vi "Set_Dark.vi"(8 "error in (no error)":errorcluster, 10 "Dark":dbl, 11 "Thorlabs_PM100D in":refnum<class "Thorlabs_PM100D.lvclass">) -> (0 "error out":errorcluster, 3 "Thorlabs_PM100D out":refnum<class "Thorlabs_PM100D.lvclass">)   [LabVIEW 2020, in "Thorlabs_PM100D.lvclass"]
uses:
  <instrlib>/Classes/Powermeter/Thorlabs_PM100D/Thorlabs_PM100D.lvclass
  <instrlib>/Classes/Powermeter/Thorlabs_PM100D/Thorlabs_PM100D.lvclass/Thorlabs_PM100D.ctl
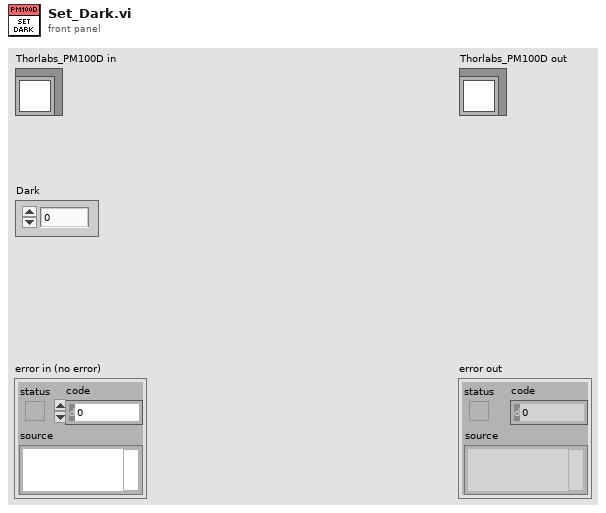
[diagram p1: front panel]
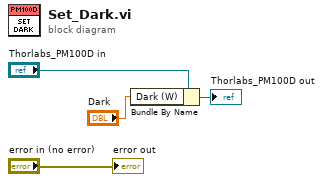
[diagram p0: block diagram]
diagram:
  n1 = Bundle By Name(cluster="Thorlabs_PM100D in", "Dark (W)"="Dark") -> (→"Thorlabs_PM100D out":refnum<class "Thorlabs_PM100D.lvclass">)
  "error out" <- "error in (no error)"
